vi "Actor Core.vi"(8 "error in":errorcluster, 11 "Generator in":refnum<class "Generator.lvclass">) -> (0 "error out":errorcluster, 3 "Actor out":refnum<class "Actor.lvclass">)   [LabVIEW 2020, in "Wrapped Actor.lvlib" / "Generator.lvclass"]
doc: "(<B>Filename</B>: Actor Framework.lvlib:Actor.lvclass:Actor Core.vi)\n\nReceives messages to the actor, reacts to them, and initiates any error handling that may shut the actor down.\n\nDescendant classes may override this VI to append parallel tasks for the actor to complete while it handles messages. Overrides use the Call Parent Class Method node."
uses:
  Generator.lvclass
  Generator.lvclass/Generator.ctl
  <vilib>/ActorFramework/Actor/Actor.lvclass
  Data Message/Data Message.lvclass
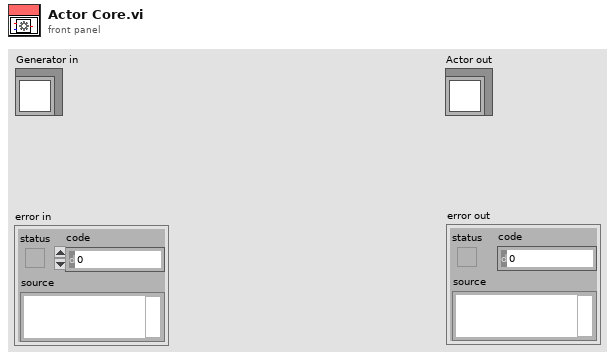
[diagram p1: front panel]
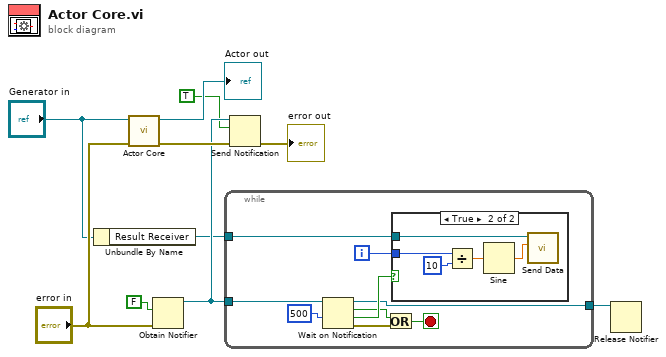
[diagram p0: block diagram]
diagram:
  n1 = Unbundle By Name("Generator in") -> ("Result Receiver"=w3:refnum<class "Message Enqueuer.lvclass">)
  n2 = call-parent "Actor Core.vi"("error in"="error in", "Actor in"="Generator in") -> ("error out"=w7:errorcluster, "Actor out"=→"Actor out":refnum<class "Actor.lvclass">)  [unwired: 8 in]
  n3 = Obtain Notifier(notification data type=FALSE, error in (no error)="error in") -> (notifier out=w6:refnum<notifier>)  [unwired: 2 in, 2 out]
  n4 = while {
    tunnel: w6 -> [w19]
    tunnel: w3 -> [w13]
    tunnel: [w11] -> w1
    i -> [w12]
    stop <- w15 stop-if-true
    n5 = Wait on Notification(notifier=w19, timeout in ms (-1)=500) -> (notifier out=w11:refnum<notifier>, notification=w16:bool, timed out?=w17:bool, error out=w14:errorcluster)  [unwired: 2 in]
    n6 = Or(x=w16, y=w14) -> (x .or. y?=w15:bool)
    n7 = case shown="True" w17 {
      tunnel: w13 -> [_ w24]
      tunnel: w12 -> [_ w23]
      frame False {
      }
      frame True {
        n8 = Divide(x=w23, y=10) -> (x/y=w22:dbl)
        n9 = Sine(x=w22) -> (sin(x)=w20:dbl)
        n10 = call "Send Data.vi"("Value"=w20, "Destination"=w24) -> ()  [unwired: 9 in, 1 out]
      }
    }
  }
  n11 = Send Notification(notification=TRUE, notifier=w6, error in (no error)=w7) -> (error out=→"error out":errorcluster)  [unwired: 1 out]
  n12 = Release Notifier(notifier=w1) -> ()  [unwired: 2 in, 3 out]
